vi "Display_Module.vi"(4 "Acquisition mode":T1, 5 "Imaging Parameter.Line Averages":u8, 6 "Y":i32=1, 7 "X":i32=2048, 8 "error in":errorcluster, 9 "Z":i32=500, 10 "Source in":T2, 11 "Angle (degrees)":sgl) -> (0 "error out":errorcluster, 2 "AIP":T2(plugin-control) caption="Image")   [LabVIEW 2018]
uses:
  <vilib>/vision/Image Controls.llb/IMAQ Image.ctl
  type defines/FFT mode.ctl
  Controls/Queue Manager Actions.ctl
  <vilib>/vision/NI_Vision_Development_Module.lvlib
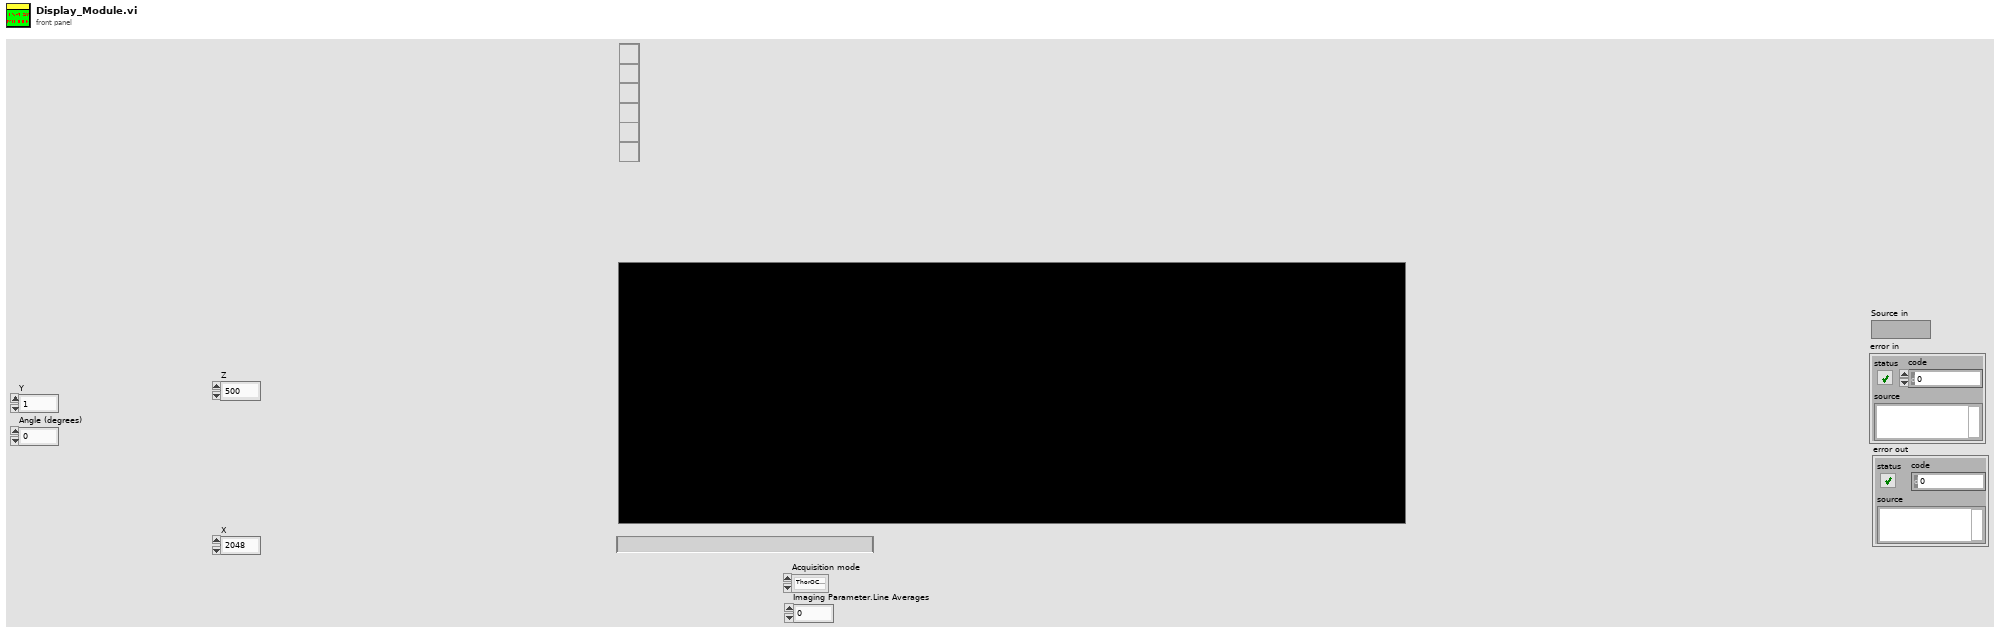
[diagram p1: front panel]
types:
  T1 = typedef "FFT mode.ctl" = enum16{"ThorOCT B line", "ThorOCT Spectral", "ThorOCT FFT", "Alazar B line", "Alazar FFT", "GPU FFT", "Alazar Spectral"}
  T2 = typedef "IMAQ Image.ctl" = refnum<image>
  T3 = typedef "Queue Manager Actions.ctl" = enum16{"Init", "Enqueue", "Enqueue All", "Preview Queue", "Dequeue", "Get Status", "Flush Queue", "Flush All Queues", "Release All Queues", "Release Queue", "Enqueue at Opposite End"}
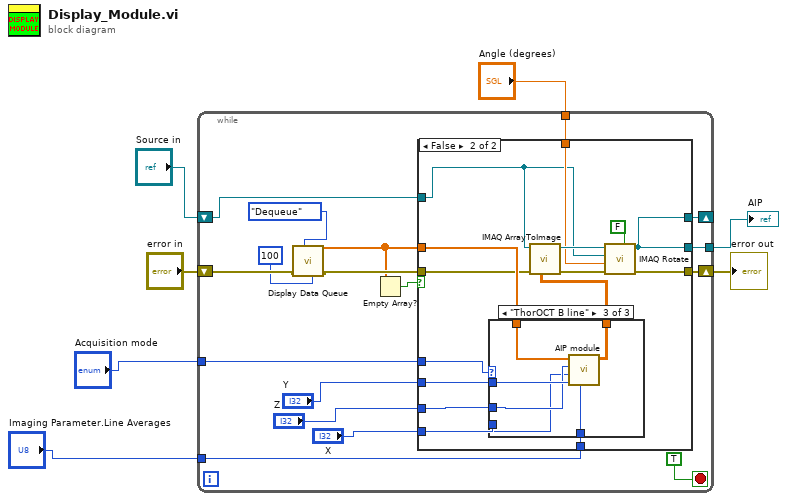
[diagram p0: block diagram]
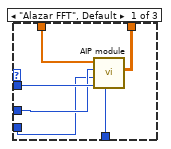
[diagram p3: hidden frame]
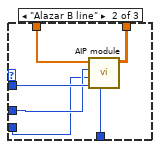
[diagram p4: hidden frame]
diagram:
  n1 = while {
    shift-right: [w24] -> w6
    shift-left: "error in" -> [w18]
    shift-right: [w21] -> _
    shift-left: "Source in" -> [w19]
    tunnel: [w20] -> w5
    tunnel: "Angle (degrees)" -> [w13]
    tunnel: "Acquisition mode" -> [w12]
    tunnel: "Imaging Parameter.Line Averages" -> [w8]
    stop <- TRUE stop-if-true
    n2 = call "Display Data Queue.vi"("timeout in ms (-1)"=100 ("time out"), "Action"=Queue_Manager_Actions."Dequeue", "error in (no error)"=w18) -> ("error out"=w17:errorcluster, "data out"=w16:sgl[])  [unwired: 5 in, 2 out]
    n3 = Empty Array?(array=w16) -> (empty?=w22:bool)
    n4 = case shown="False" w22 {
      tunnel: w17 -> [w26 w29]
      tunnel: [w26 w41] -> w24
      tunnel: w16 -> [_ w36]
      tunnel: [w25 w37] -> w21
      tunnel: [w25 w37] -> w20
      tunnel: w19 -> [w25 w28]
      tunnel: w13 -> [_ w35]
      tunnel: w12 -> [_ w27]
      tunnel: "Y" -> [_ w33]
      tunnel: "Z" -> [_ w32]
      tunnel: "X" -> [_ w31]
      tunnel: w8 -> [_ w30]
      frame True {
      }
      frame False {
        n5 = case shown="\"ThorOCT B line\"" w27 {
          tunnel: w36 -> [w47 w53 w59]
          tunnel: [w46 w48 w54] -> w34
          tunnel: w33 -> [w45 w52 w58]
          tunnel: w32 -> [w44 w51 w57]
          tunnel: w31 -> [w43 w50 w56]
          tunnel: w30 -> [w42 w49 w55]
          frame "Alazar FFT", Default {
            n6 = call "AIP module.vi"("Imaging Parameter.Line Averages"=w42, "Y"=w45, "X"=w43, "Z"=w44, "3D volume"=w47) -> ("AIP"=w46:sgl[][])  [unwired: 5 in, 1 out]
          }
          frame "Alazar B line" {
            n7 = call "AIP module.vi"("Imaging Parameter.Line Averages"=w49, "Y"=w52, "X"=w50, "Z"=w51, "3D volume"=w53) -> ("Bline"=w48:dbl[][])  [unwired: 5 in, 1 out]
          }
          frame "ThorOCT B line" {
            n8 = call "AIP module.vi"("Imaging Parameter.Line Averages"=w55, "Y"=w58, "X"=w56, "Z"=w57, "3D volume"=w59) -> ("Bline"=w54:dbl[][])  [unwired: 5 in, 1 out]
          }
        }
        n9 = call "IMAQ ArrayToImage"("Image Pixels (Float)"=w34, "error in (no error)"=w29, "Image"=w28) -> ("error out"=w39:errorcluster, "Image Out"=w40:T2)  [unwired: 7 in]
        n10 = call "IMAQ Rotate"("Maintain Size"=FALSE, "error in (no error)"=w39, "Angle (degrees)"=w35, "Image Dst"=w28, "Image Src"=w40) -> ("error out"=w41:errorcluster, "Image Dst Out"=w37:T2)  [unwired: 5 in]
      }
    }
  }
  "error out" <- w6
  "AIP" <- w5
